vi "File.Rotate.Config Dialog.vi"(8 "error in (no error)":errorcluster, 11 "File.Rotate in":refnum<class "File.Rotate.lvclass">) -> (0 "error out":errorcluster, 1 "OK":bool, 2 "Rotation Config":T1[](array[typedef]), 3 "File.Rotate out":refnum<class "File.Rotate.lvclass">)   [LabVIEW 2024, in "EQMF.lvlib" / "File Utils.lvlib" / "File.Rotate.lvclass"]
uses:
  File.Rotate.lvclass
  File.Rotate.Rotation Task Item.ctl
  File.Rotate.lvclass/File.Rotate.ctl
panel:
  out "Tab Control":enum32{"Input", "Dialog", "Output"}(tab)=enum."Dialog"
  in  "Cancel Button":bool
  in  "OK Button":bool
  in  "Rotation Config":T1[](array[typedef])
  # "File Rotation Setup"
  # "Name/Interval                                                                                             Folder and Max Counts"
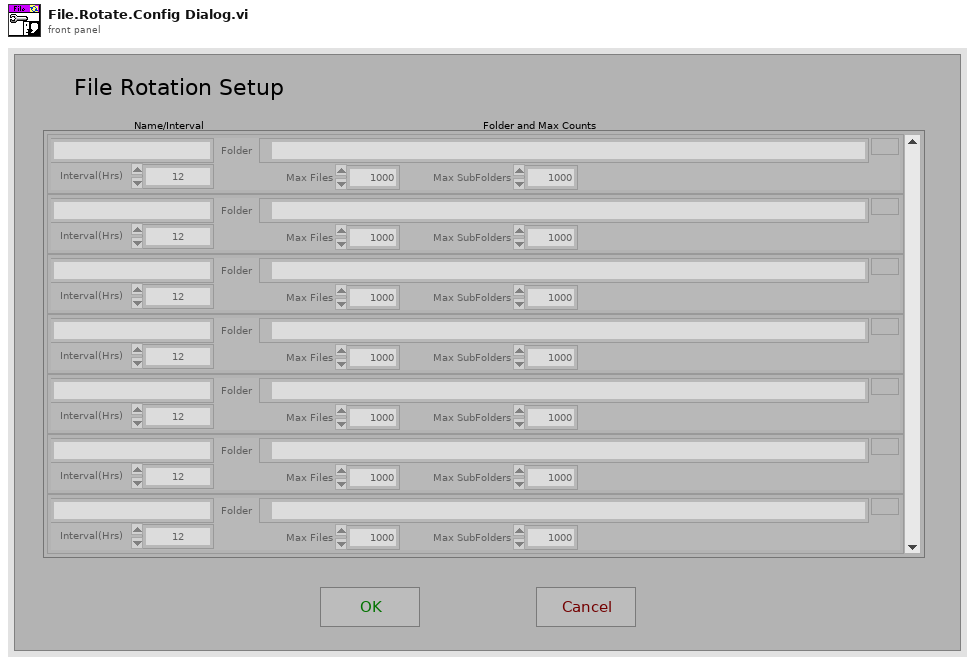
[diagram p1: front panel]
types:
  T1 = typedef "EQMF.lvlib/File Utils.lvlib/File.Rotate.lvclass/File.Rotate.Rotation Task Item.ctl" = cluster{"Name":string, "Interval":dbl, "Folder":path, "Max Files":i32, "Max SubFolders":i32, "LastRotate":timestamp, "Error":bool, "Status":string}
  T2 = enum32{"Invalid", "Standard", "Closed", "Hidden", "Minimized", "Maximized"}
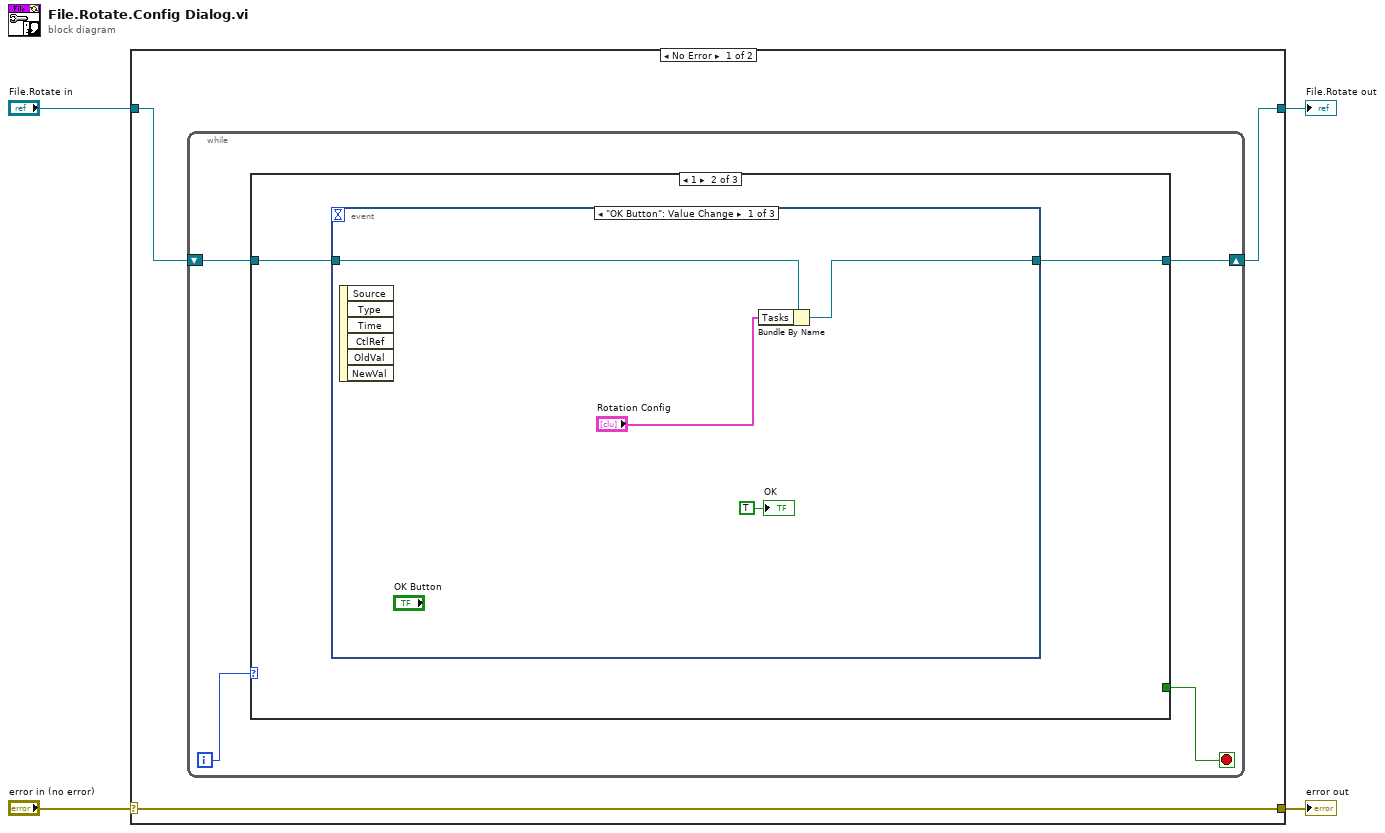
[diagram p0: block diagram]
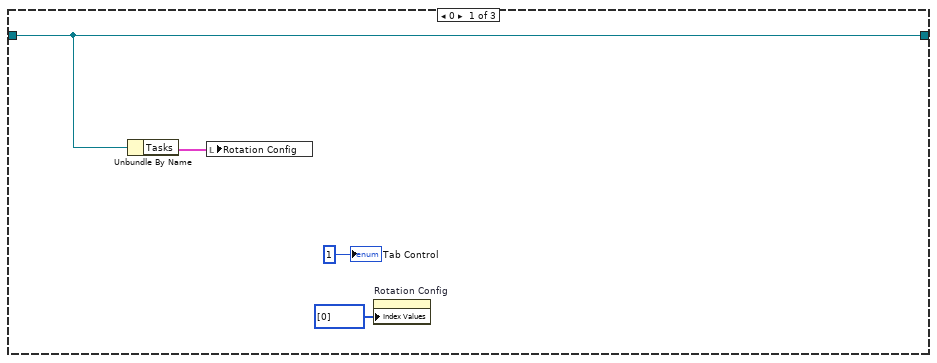
[diagram p2: hidden frame]
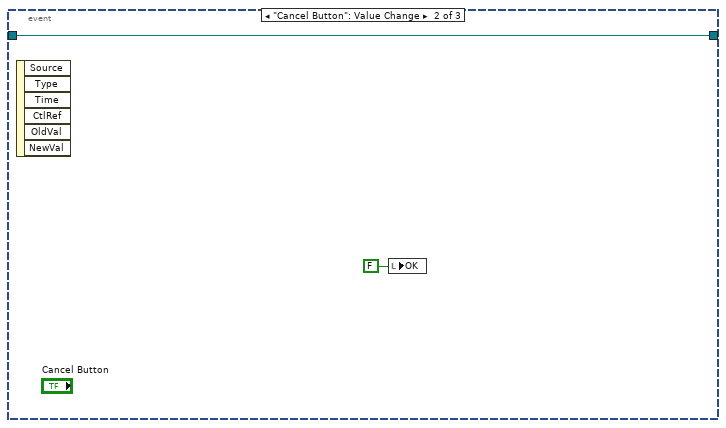
[diagram p3: hidden frame]
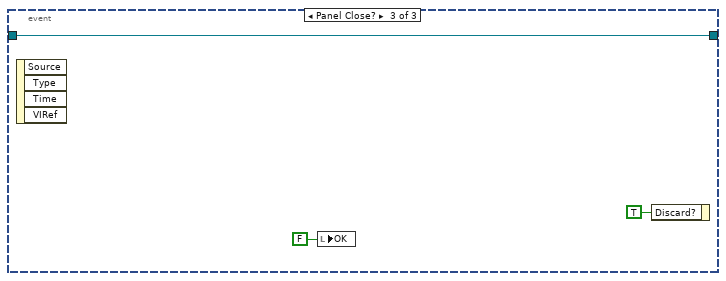
[diagram p4: hidden frame]
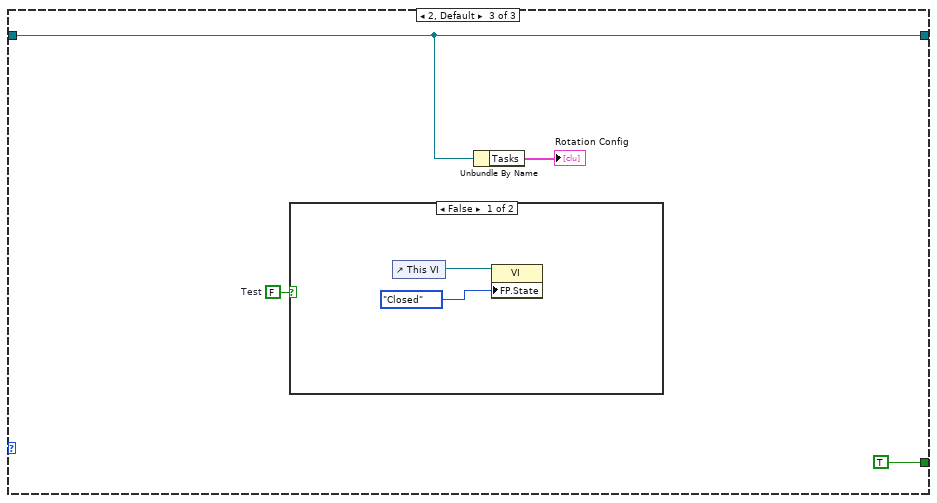
[diagram p5: hidden frame]
diagram:
  n1 = case shown="No Error" "error in (no error)" {
    selector: "error in (no error)" -> [w7 w34]
    tunnel: [w7 w34] -> w3
    tunnel: [w5 w33] -> w1
    tunnel: "File.Rotate in" -> [w6 w33]
    frame No Error {
      n2 = while {
        shift-right: [w9] -> w5
        shift-left: w6 -> [w11]
        i -> [w10]
        stop <- w8 stop-if-true
        n3 = case shown="1" w10 {
          tunnel: w11 -> [w12 w17 w28]
          tunnel: [w12 w16 w28] -> w9
          tunnel: [_ _ TRUE] -> w8
          frame 0 {
            n4 = Unbundle By Name(w12) -> ("Tasks"=w13:T1[])
            n5 = local write "Rotation Config"(w13) -> ()
            n6 = property on="Rotation Config" class="Arr (strict)"("Index Values"=u32[] [0]) -> ()  [unwired: 2 in, 2 out]
            "Tab Control" <- 1
          }
          frame 1 {
            n7 = event shown="[0] \"OK Button\": Value Change" {
              selector: _ -> [_ _ _]
              dyn-events: _ -> [_ _ _]
              timeout: _ -> [_ _ _]
              tunnel: w17 -> [w20 w22 w25]
              tunnel: [w19 w22 w25] -> w16
              event "OK Button": Value Change {
                n8 = event-data() -> ()  [unwired: 1 in, 6 out]
                n9 = Bundle By Name(cluster=w20, "Tasks"="Rotation Config") -> (w19:refnum<class "File.Rotate.lvclass">)
                "OK" <- TRUE ("OK")
              }
              event "Cancel Button": Value Change {
                n10 = event-data() -> ()  [unwired: 1 in, 6 out]
                n11 = local write "OK"(FALSE ("OK")) -> ()
              }
              event Panel Close? {
                n12 = event-data() -> ()  [unwired: 1 in, 4 out]
                n13 = local write "OK"(FALSE ("OK")) -> ()
                n14 = event-data("Discard?"=TRUE) -> ()  [unwired: 1 in, 1 out]
              }
            }
          }
          frame 2, Default {
            w30 = FALSE  # Test
            n15 = case shown="False" w30 {
              frame False {
                n16 = control-ref of="This VI"() -> (w32:refnum<vi>)
                n17 = property class="VI"(reference=w32, "FP.State"=T2."Closed" ("Front Panel Window:State")) -> ()  [unwired: 1 in, 2 out]
              }
              frame True {
              }
            }
            n18 = Unbundle By Name(w28) -> ("Tasks"=→"Rotation Config":T1[])
          }
        }
      }
    }
    frame Error {
    }
  }
  "error out" <- w3
  "File.Rotate out" <- w1
